vi "GetInsideTerminals.vi"(6 "error in":errorcluster, 9 "RightShiftRegister in":refnum<class "RightShiftRegister.lvclass">) -> (0 "error out":errorcluster, 3 "RightShiftRegister out":refnum<class "RightShiftRegister.lvclass">, 4 "Terminals":refnum<class "Terminal.lvclass">[](array[class]))   [LabVIEW 2014, in "Raspberry Pi Compatible Compiler for LabVIEW.lvlib" / "RightShiftRegister.lvclass"]
uses:
  RightShiftRegister.lvclass
  Terminal/Terminal.lvclass
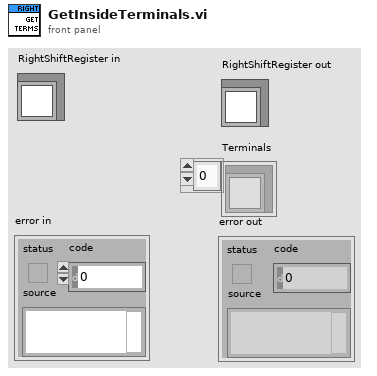
[diagram p1: front panel]
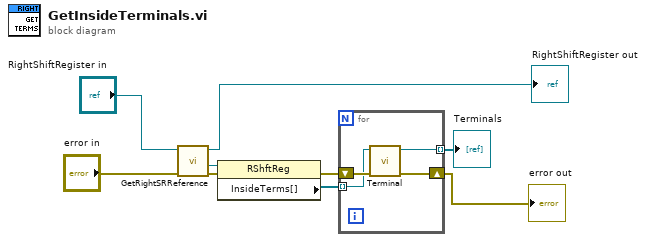
[diagram p0: block diagram]
diagram:
  n1 = call "GetRightSRReference.vi"("error in"="error in", "ShiftRegister in"="RightShiftRegister in") -> ("error out"=w5:errorcluster, "reference out"=w6:refnum<vi>, "ShiftRegister out"=→"RightShiftRegister out":refnum<class "RightShiftRegister.lvclass">)  [unwired: 7 in]
  n2 = property class="RShftReg"(reference=w6, error in=w5) -> (error out=w4:errorcluster, "InsideTerms[]"=w3:refnum<vi>[])  [unwired: 1 out]
  n3 = for {
    tunnel: w3 -> [w12] mode=indexing
    shift-right: [w11] -> w1
    shift-left: w4 -> [w13]
    tunnel: [w10] -> w2 mode=indexing
    n4 = call "Terminal.vi"("error in"=w13, "refnum"=w12) -> ("error out"=w11:errorcluster, "terminal"=w10:refnum<class "Terminal.lvclass">)  [unwired: 8 in]
  }
  "error out" <- w1
  "Terminals" <- w2
